vi "set_data_for_channel.vi"(8 "error in (no error)":errorcluster, 10 "data":dbl[](array[numeric]), 11 "GenericWriteSignals in":refnum<class "SignalWriterDL101123SoundCard.lvclass">) -> (0 "error out":errorcluster, 3 "GenericWriteSignals out":refnum<class "SignalWriterDL101123SoundCard.lvclass">)   [LabVIEW 2010, in "SignalWriterDL101123SoundCard.lvclass"]
uses:
  SignalWriterDL101123SoundCard.lvclass
  SignalWriterDL101123SoundCard.lvclass/SignalWriterDL101123SoundCard.ctl
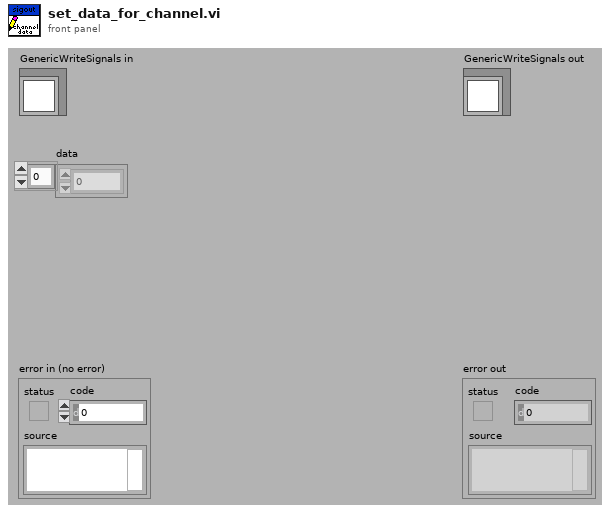
[diagram p1: front panel]
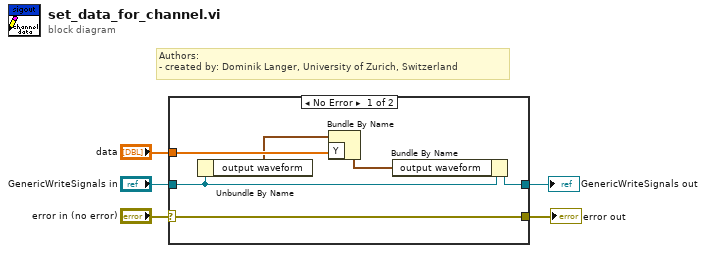
[diagram p0: block diagram]
diagram:
  # "Authors: \n- created by: Dominik Langer, University of Zurich, Switzerland"
  n1 = case shown="No Error" "error in (no error)" {
    selector: "error in (no error)" -> [w11 w12]
    tunnel: "GenericWriteSignals in" -> [w7 w13]
    tunnel: [w11 w12] -> w3
    tunnel: [w9 w13] -> w2
    tunnel: "data" -> [w10 _]
    frame No Error {
      n2 = Unbundle By Name(w7) -> ("output waveform"=w6:waveform(dbl))
      n3 = Bundle By Name(cluster=w6, "Y"=w10) -> (w8:waveform(dbl))
      n4 = Bundle By Name(cluster=w7, "output waveform"=w8) -> (w9:refnum<class "SignalWriterDL101123SoundCard.lvclass">)
    }
    frame Error {
    }
  }
  "error out" <- w3
  "GenericWriteSignals out" <- w2
